vi "Close All Blanks.vi"(8 "error in (no error)":errorcluster, 11 "2DArrayManager in":refnum<class "2DArrayManager.lvclass">) -> (0 "error out":errorcluster, 3 "2DArrayManager out":refnum<class "2DArrayManager.lvclass">)   [LabVIEW 2020, in "OOPanel.lvlib" / "2DArrayManager.lvclass"]
uses:
  2DArrayManager.lvclass
  2DArrayManager.lvclass/2DArrayManager.ctl
  2DPanelBlank/2DPanelBlank.lvclass
  C:/dev/lv20CE/lv-oopanel/OOPanel/Panel/Panel.lvclass
  Manager/Manager.lvclass
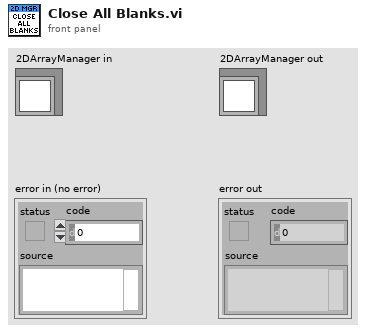
[diagram p1: front panel]
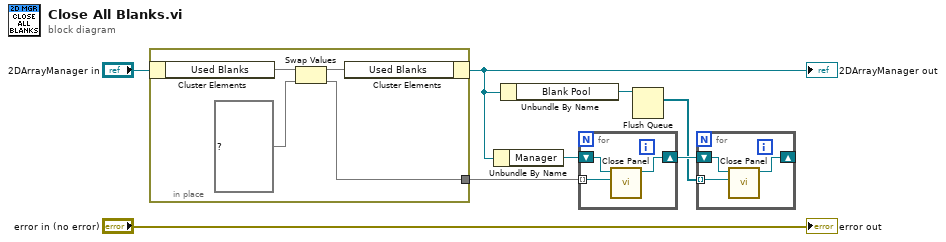
[diagram p0: block diagram]
diagram:
  n1 = in-place {
    in-place-border: [w11] -> w6
    n2 = in-place-cluster #1("2DArrayManager in") -> ("Used Blanks"=w10:set{refnum<class "2DPanelBlank.lvclass">})
    n3 = Swap Values(12:w10, 14:set{refnum<class "2DPanelBlank.lvclass">} {} ("UI Refs.Used Blanks")) -> (1:w12:set{refnum<class "2DPanelBlank.lvclass">}, 3:w11:set{refnum<class "2DPanelBlank.lvclass">})  [unwired: 1 in]
    n4 = in-place-cluster #1("Used Blanks"=w12) -> (w3:refnum<class "2DArrayManager.lvclass">)
  }
  "2DArrayManager out" <- w3
  n5 = Unbundle By Name(w3) -> ("Manager"=w5:refnum<class "Manager.lvclass">)
  n6 = Unbundle By Name(w3) -> ("Blank Pool"=w2:refnum<queue>)
  n7 = for {
    tunnel: w6 -> [w15] mode=indexing
    shift-right: [w13] -> w4
    shift-left: w5 -> [w14]
    n8 = call "Close Panel.vi"("Panel"=w15, "Manager in"=w14) -> ("Manager out"=w13:refnum<class "Manager.lvclass">)  [unwired: 8 in, 1 out]
  }
  n9 = Flush Queue(queue=w2) -> (remaining elements=w1:refnum<class "2DPanelBlank.lvclass">[])  [unwired: 1 in, 2 out]
  n10 = for {
    tunnel: w1 -> [w18] mode=indexing
    shift-right: [w16] -> _
    shift-left: w4 -> [w17]
    n11 = call "Close Panel.vi"("Panel"=w18, "Manager in"=w17) -> ("Manager out"=w16:refnum<class "Manager.lvclass">)  [unwired: 8 in, 1 out]
  }
  "error out" <- "error in (no error)"
